vi "Begin Swerve Drive.vi"   [LabVIEW 2018]
uses:
  <vilib>/Rock Robotics/SystemInterfaces/DIO/FPGA_DIOPWMChannel.ctl
  <vilib>/Rock Robotics/SystemInterfaces/AI/FPGA_AIChannel.ctl
  <vilib>/Rock Robotics/SystemInterfaces/DIO/FPGA_DIOChannel.ctl
  <vilib>/Rock Robotics/WPI/RobotDrive/WPI_RobotDriveOpen4MotorWithTalon.vi
  <vilib>/Rock Robotics/WPI/Counter/WPI_CounterDigitalInputToDigitalSource.vi
types:
  T1 = typedef "FPGA_DIOChannel.ctl" = enum8{"DIO 0", "DIO 1", "DIO 2", "DIO 3", "DIO 4", "DIO 5", "DIO 6", "DIO 7", "DIO 8", "DIO 9", "DIO MXP 0", "DIO MXP 1", "DIO MXP 2", "DIO MXP 3", "DIO MXP 4", "DIO MXP 5", "DIO MXP 6", "DIO MXP 7", "DIO MXP 8", "DIO MXP 9", "DIO MXP 10", "DIO MXP 11", "DIO MXP 12", "DIO MXP 13", "DIO MXP 14", "DIO MXP 15", "SPI Port CS1", "SPI Port CS2", "SPI Port CS3", "SPI Port MISO", "SPI Port MOSI", "Invalid"}
  T2 = typedef "FPGA_AIChannel.ctl" = enum8{"AI 0", "AI 1", "AI 2", "AI 3", "AI MXP 0", "AI MXP 1", "AI MXP 2", "AI MXP 3", "Invalid"}
  T3 = typedef "FPGA_DIOPWMChannel.ctl" = enum8{"PWM 0", "PWM 1", "PWM 2", "PWM 3", "PWM 4", "PWM 5", "PWM 6", "PWM 7", "PWM 8", "PWM 9", "PWM MXP 0", "PWM MXP 1", "PWM MXP 2", "PWM MXP 3", "PWM MXP 4", "PWM MXP 5", "PWM MXP 6", "PWM MXP 7", "PWM MXP 8", "PWM MXP 9", "Invalid"}
  T4 = typedef "WPI_RobotDriveDevRef.ctl" = cluster{"DevStatus":errorcluster, "Motors[]":T5[], "Square Inputs":bool, "Max Output":dbl}
  T5 = typedef "WPI_MotorControlDeviceRef.ctl" = cluster{"DeviceStatus":errorcluster, "Type":T6, "PWM":cluster{"PWM Channel":T3, "DeadBand":T7}, "CAN":cluster{"Device Number":u8, "SetOutput VI Ref":variant, "GetOutput VI Ref":variant, "Enable VI Ref":variant, "Disable VI Ref":variant, "Data":variant}, "Invert":bool, "DIO PWM":cluster{"PWM \"Enable\" Channel":T3, "DIOChannel":T1, "PWM Rate":dbl}}
  T6 = typedef "WPI_MotorControlType.ctl" = enum16{"PWM", "CAN", "DIO PWM"}
  T7 = typedef "WPI_PWMDeadband.ctl" = cluster{"Name":string, "maxPositivePwm":i32, "minPositivePwm":i32, "centerPwm":i32, "maxNegativePwm":i32, "minNegativePwm":i32, "angularRange":u16}
  T8 = typedef "WPI_AnalogChannelDevRef.ctl" = cluster{"DevStatus":errorcluster, "Analog Channel":T2}
  T9 = typedef "WPI_DigitalInputDevRef.ctl" = cluster{"DevStatus":errorcluster, "DIO Channel":T1}
  T10 = typedef "FPGA_CounterEncoderSourceConvertionLVSourceType.ctl" = cluster{"DevStatus":errorcluster, "AnalogTriggerMode?":bool, "DigitalMode":cluster{"DIO Channel":T11}, "AnalogTriggerMode":cluster{"AnalogTriggerIndex":T12, "OutputType":T13}}
  T11 = typedef "FPGA_DIODigitalSourceChannel.ctl" = enum8{"DIO 0", "DIO 1", "DIO 2", "DIO 3", "DIO 4", "DIO 5", "DIO 6", "DIO 7", "DIO 8", "DIO 9", "DIO MXP 0", "DIO MXP 1", "DIO MXP 2", "DIO MXP 3", "DIO MXP 4", "DIO MXP 5", "DIO MXP 6", "DIO MXP 7", "DIO MXP 8", "DIO MXP 9", "DIO MXP 10", "DIO MXP 11", "DIO MXP 12", "DIO MXP 13", "DIO MXP 14", "DIO MXP 15", "SPI Port CS1", "SPI Port CS2", "SPI Port CS3", "SPI Port MISO", "SPI Port MOSI", "Disabled"}
  T12 = typedef "FPGA_AnalogTriggerIndex.ctl" = enum8{"Trig 0", "Trig 1", "Trig 2", "Trig 3", "Trig 4", "Trig 5", "Trig 6", "Trig 7", "Invalid"}
  T13 = typedef "FPGA_AnalogTriggerOutType.ctl" = enum16{"InWindow", "TriggerState", "Rising", "Falling"}
  T14 = typedef "WPI_EncoderDevRef.ctl" = cluster{"DevStatus":errorcluster, "EncoderIndex":T15, "CounterIndex":T16, "DistancePerCount":dbl, "Decoding Type":T17}
  T15 = typedef "FPGA_EncoderIdx.ctl" = enum8{"Enc 0", "Enc 1", "Enc 2", "Enc 3", "Enc 4", "Enc 5", "Enc 6", "Enc 7", "Invalid"}
  T16 = typedef "FPGA_CounterCtrSystemIndex.ctl" = enum8{"Ctr 0", "Ctr 1", "Ctr 2", "Ctr 3", "Ctr 4", "Ctr 5", "Ctr 6", "Ctr 7", "Invalid"}
  T17 = typedef "WPI_EncoderType.ctl" = enum16{"1x", "2x", "4x"}
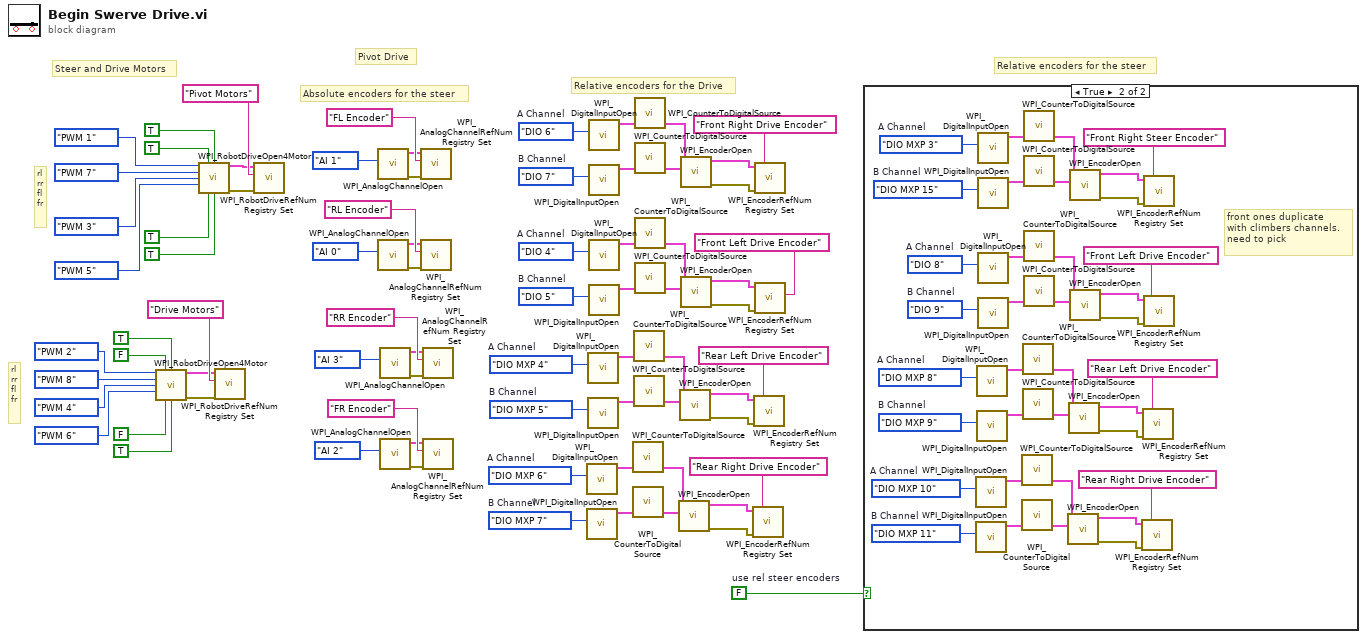
[diagram p0: block diagram]
diagram:
  w1 = FALSE  # use rel steer encoders
  w10 = FPGA_DIOChannel."DIO MXP 7"  # B Channel
  w9 = FPGA_DIOChannel."DIO MXP 6"  # A Channel
  w19 = FPGA_DIOChannel."DIO MXP 5"  # B Channel
  w18 = FPGA_DIOChannel."DIO MXP 4"  # A Channel
  w28 = FPGA_DIOChannel."DIO 5"  # B Channel
  w27 = FPGA_DIOChannel."DIO 4"  # A Channel
  w37 = FPGA_DIOChannel."DIO 7"  # B Channel
  w36 = FPGA_DIOChannel."DIO 6"  # A Channel
  # "Steer and Drive Motors"
  # "Absolute encoders for the steer"
  # "Relative encoders for the Drive"
  # "Relative encoders for the steer"
  # "Pivot Drive"
  # "rl\nrr\nfl\nfr"
  # "rl\nrr\nfl\nfr"
  n1 = call-poly <vilib>:"WPI_RobotDriveOpen4Motor.vi"("Rear Left Motor"=FPGA_DIOPWMChannel."PWM 2", "Rear Left Motor Inverted"=FALSE, "Rear Right Motor Inverted"=TRUE, "Rear Right Motor"=FPGA_DIOPWMChannel."PWM 8", "Front Left Motor"=FPGA_DIOPWMChannel."PWM 4", "Front Right Motor"=FPGA_DIOPWMChannel."PWM 6", "Front Left Motor Inverted"=FALSE, "Front Right Motor Inverted"=TRUE) -> ("RobotDriveDevRef"=w50:T4, "error out"=w49:errorcluster)  [unwired: 6 in]
  n2 = call-poly <vilib>:"WPI_RobotDriveOpen4Motor.vi"("Rear Left Motor"=FPGA_DIOPWMChannel."PWM 1", "Rear Left Motor Inverted"=TRUE, "Rear Right Motor Inverted"=TRUE, "Rear Right Motor"=FPGA_DIOPWMChannel."PWM 7", "Front Left Motor"=FPGA_DIOPWMChannel."PWM 3", "Front Right Motor"=FPGA_DIOPWMChannel."PWM 5", "Front Left Motor Inverted"=TRUE, "Front Right Motor Inverted"=TRUE) -> ("RobotDriveDevRef"=w39:T4, "error out"=w38:errorcluster)  [unwired: 6 in]
  n3 = call <vilib>:"WPI_RobotDriveRefNum Registry Set.vi"("error in (no error)"=w49, "refnum name"="Drive Motors", "RobotDriveDevRef"=w50) -> ()  [unwired: 7 in, 2 out]
  n4 = call <vilib>:"WPI_RobotDriveRefNum Registry Set.vi"("error in (no error)"=w38, "refnum name"="Pivot Motors", "RobotDriveDevRef"=w39) -> ()  [unwired: 7 in, 2 out]
  n5 = call <vilib>:"WPI_AnalogChannelOpen.vi"("Analog Channel"=FPGA_AIChannel."AI 1") -> ("error out"=w64:errorcluster, "AIDeviceRef"=w65:T8)  [unwired: 9 in]
  n6 = call <vilib>:"WPI_AnalogChannelOpen.vi"("Analog Channel"=FPGA_AIChannel."AI 0") -> ("error out"=w60:errorcluster, "AIDeviceRef"=w61:T8)  [unwired: 9 in]
  n7 = call <vilib>:"WPI_AnalogChannelOpen.vi"("Analog Channel"=FPGA_AIChannel."AI 3") -> ("error out"=w72:errorcluster, "AIDeviceRef"=w73:T8)  [unwired: 9 in]
  n8 = call <vilib>:"WPI_AnalogChannelOpen.vi"("Analog Channel"=FPGA_AIChannel."AI 2") -> ("error out"=w68:errorcluster, "AIDeviceRef"=w69:T8)  [unwired: 9 in]
  n9 = call <vilib>:"WPI_AnalogChannelRefNum Registry Set.vi"("error in (no error)"=w64, "refnum name"="FL Encoder", "AIDeviceRef"=w65) -> ()  [unwired: 7 in, 2 out]
  n10 = call <vilib>:"WPI_AnalogChannelRefNum Registry Set.vi"("error in (no error)"=w60, "refnum name"="RL Encoder", "AIDeviceRef"=w61) -> ()  [unwired: 7 in, 2 out]
  n11 = call <vilib>:"WPI_AnalogChannelRefNum Registry Set.vi"("error in (no error)"=w72, "refnum name"="RR Encoder", "AIDeviceRef"=w73) -> ()  [unwired: 7 in, 2 out]
  n12 = call <vilib>:"WPI_AnalogChannelRefNum Registry Set.vi"("error in (no error)"=w68, "refnum name"="FR Encoder", "AIDeviceRef"=w69) -> ()  [unwired: 7 in, 2 out]
  n13 = call <vilib>:"WPI_DigitalInputOpen.vi"("DIO Channel"=w9) -> ("DigitalInputDevRef"=w6:T9)  [unwired: 1 in, 9 out]
  n14 = call <vilib>:"WPI_DigitalInputOpen.vi"("DIO Channel"=w10) -> ("DigitalInputDevRef"=w7:T9)  [unwired: 1 in, 9 out]
  n15 = call <vilib>:"WPI_DigitalInputOpen.vi"("DIO Channel"=w18) -> ("DigitalInputDevRef"=w15:T9)  [unwired: 1 in, 9 out]
  n16 = call <vilib>:"WPI_DigitalInputOpen.vi"("DIO Channel"=w19) -> ("DigitalInputDevRef"=w16:T9)  [unwired: 1 in, 9 out]
  n17 = call <vilib>:"WPI_DigitalInputOpen.vi"("DIO Channel"=w36) -> ("DigitalInputDevRef"=w33:T9)  [unwired: 1 in, 9 out]
  n18 = call <vilib>:"WPI_DigitalInputOpen.vi"("DIO Channel"=w37) -> ("DigitalInputDevRef"=w34:T9)  [unwired: 1 in, 9 out]
  n19 = call <vilib>:"WPI_DigitalInputOpen.vi"("DIO Channel"=w27) -> ("DigitalInputDevRef"=w24:T9)  [unwired: 1 in, 9 out]
  n20 = call <vilib>:"WPI_DigitalInputOpen.vi"("DIO Channel"=w28) -> ("DigitalInputDevRef"=w25:T9)  [unwired: 1 in, 9 out]
  n21 = call-poly <vilib>:"WPI_CounterToDigitalSource.vi"("DigitalInputDevRef"=w6) -> ("Digital Source"=w5:T10)  [unwired: 6 out]
  n22 = call-poly <vilib>:"WPI_CounterToDigitalSource.vi"("DigitalInputDevRef"=w7) -> ("Digital Source"=w8:T10)  [unwired: 6 out]
  n23 = call-poly <vilib>:"WPI_CounterToDigitalSource.vi"("DigitalInputDevRef"=w15) -> ("Digital Source"=w14:T10)  [unwired: 6 out]
  n24 = call-poly <vilib>:"WPI_CounterToDigitalSource.vi"("DigitalInputDevRef"=w16) -> ("Digital Source"=w17:T10)  [unwired: 6 out]
  n25 = call-poly <vilib>:"WPI_CounterToDigitalSource.vi"("DigitalInputDevRef"=w33) -> ("Digital Source"=w32:T10)  [unwired: 6 out]
  n26 = call-poly <vilib>:"WPI_CounterToDigitalSource.vi"("DigitalInputDevRef"=w34) -> ("Digital Source"=w35:T10)  [unwired: 6 out]
  n27 = call-poly <vilib>:"WPI_CounterToDigitalSource.vi"("DigitalInputDevRef"=w24) -> ("Digital Source"=w23:T10)  [unwired: 6 out]
  n28 = call-poly <vilib>:"WPI_CounterToDigitalSource.vi"("DigitalInputDevRef"=w25) -> ("Digital Source"=w26:T10)  [unwired: 6 out]
  n29 = call <vilib>:"WPI_EncoderOpen.vi"("BSource"=w8, "ASource"=w5) -> ("error out"=w3:errorcluster, "EncoderDevRef"=w4:T14)  [unwired: 6 in, 2 out]
  n30 = call <vilib>:"WPI_EncoderOpen.vi"("BSource"=w17, "ASource"=w14) -> ("error out"=w12:errorcluster, "EncoderDevRef"=w13:T14)  [unwired: 6 in, 2 out]
  n31 = call <vilib>:"WPI_EncoderOpen.vi"("BSource"=w35, "ASource"=w32) -> ("error out"=w30:errorcluster, "EncoderDevRef"=w31:T14)  [unwired: 6 in, 2 out]
  n32 = call <vilib>:"WPI_EncoderOpen.vi"("BSource"=w26, "ASource"=w23) -> ("error out"=w21:errorcluster, "EncoderDevRef"=w22:T14)  [unwired: 6 in, 2 out]
  n33 = call <vilib>:"WPI_EncoderRefNum Registry Set.vi"("error in (no error)"=w3, "refnum name"="Rear Right Drive Encoder", "EncoderDevRef"=w4) -> ()  [unwired: 7 in, 2 out]
  n34 = call <vilib>:"WPI_EncoderRefNum Registry Set.vi"("error in (no error)"=w12, "refnum name"="Rear Left Drive Encoder", "EncoderDevRef"=w13) -> ()  [unwired: 7 in, 2 out]
  n35 = call <vilib>:"WPI_EncoderRefNum Registry Set.vi"("error in (no error)"=w30, "refnum name"="Front Right Drive Encoder", "EncoderDevRef"=w31) -> ()  [unwired: 7 in, 2 out]
  n36 = call <vilib>:"WPI_EncoderRefNum Registry Set.vi"("error in (no error)"=w21, "refnum name"="Front Left Drive Encoder", "EncoderDevRef"=w22) -> ()  [unwired: 7 in, 2 out]
  n37 = case shown="True" w1 {
    frame False {
    }
    frame True {
      w103 = FPGA_DIOChannel."DIO MXP 11"  # B Channel
      w104 = FPGA_DIOChannel."DIO MXP 10"  # A Channel
      w94 = FPGA_DIOChannel."DIO MXP 9"  # B Channel
      w95 = FPGA_DIOChannel."DIO MXP 8"  # A Channel
      w85 = FPGA_DIOChannel."DIO 9"  # B Channel
      w86 = FPGA_DIOChannel."DIO 8"  # A Channel
      w76 = FPGA_DIOChannel."DIO MXP 15"  # B Channel
      w77 = FPGA_DIOChannel."DIO MXP 3"  # A Channel
      # "front ones duplicate\nwith climbers channels.\nneed to pick"
      n38 = call <vilib>:"WPI_DigitalInputOpen.vi"("DIO Channel"=w104) -> ("DigitalInputDevRef"=w107:T9)  [unwired: 1 in, 9 out]
      n39 = call <vilib>:"WPI_DigitalInputOpen.vi"("DIO Channel"=w103) -> ("DigitalInputDevRef"=w106:T9)  [unwired: 1 in, 9 out]
      n40 = call <vilib>:"WPI_DigitalInputOpen.vi"("DIO Channel"=w95) -> ("DigitalInputDevRef"=w98:T9)  [unwired: 1 in, 9 out]
      n41 = call <vilib>:"WPI_DigitalInputOpen.vi"("DIO Channel"=w94) -> ("DigitalInputDevRef"=w97:T9)  [unwired: 1 in, 9 out]
      n42 = call <vilib>:"WPI_DigitalInputOpen.vi"("DIO Channel"=w77) -> ("DigitalInputDevRef"=w80:T9)  [unwired: 1 in, 9 out]
      n43 = call <vilib>:"WPI_DigitalInputOpen.vi"("DIO Channel"=w76) -> ("DigitalInputDevRef"=w79:T9)  [unwired: 1 in, 9 out]
      n44 = call <vilib>:"WPI_DigitalInputOpen.vi"("DIO Channel"=w86) -> ("DigitalInputDevRef"=w89:T9)  [unwired: 1 in, 9 out]
      n45 = call <vilib>:"WPI_DigitalInputOpen.vi"("DIO Channel"=w85) -> ("DigitalInputDevRef"=w88:T9)  [unwired: 1 in, 9 out]
      n46 = call-poly <vilib>:"WPI_CounterToDigitalSource.vi"("DigitalInputDevRef"=w107) -> ("Digital Source"=w108:T10)  [unwired: 6 out]
      n47 = call-poly <vilib>:"WPI_CounterToDigitalSource.vi"("DigitalInputDevRef"=w106) -> ("Digital Source"=w105:T10)  [unwired: 6 out]
      n48 = call-poly <vilib>:"WPI_CounterToDigitalSource.vi"("DigitalInputDevRef"=w98) -> ("Digital Source"=w99:T10)  [unwired: 6 out]
      n49 = call-poly <vilib>:"WPI_CounterToDigitalSource.vi"("DigitalInputDevRef"=w97) -> ("Digital Source"=w96:T10)  [unwired: 6 out]
      n50 = call-poly <vilib>:"WPI_CounterToDigitalSource.vi"("DigitalInputDevRef"=w80) -> ("Digital Source"=w81:T10)  [unwired: 6 out]
      n51 = call-poly <vilib>:"WPI_CounterToDigitalSource.vi"("DigitalInputDevRef"=w79) -> ("Digital Source"=w78:T10)  [unwired: 6 out]
      n52 = call-poly <vilib>:"WPI_CounterToDigitalSource.vi"("DigitalInputDevRef"=w89) -> ("Digital Source"=w90:T10)  [unwired: 6 out]
      n53 = call-poly <vilib>:"WPI_CounterToDigitalSource.vi"("DigitalInputDevRef"=w88) -> ("Digital Source"=w87:T10)  [unwired: 6 out]
      n54 = call <vilib>:"WPI_EncoderOpen.vi"("BSource"=w105, "ASource"=w108) -> ("error out"=w110:errorcluster, "EncoderDevRef"=w109:T14)  [unwired: 6 in, 2 out]
      n55 = call <vilib>:"WPI_EncoderOpen.vi"("BSource"=w96, "ASource"=w99) -> ("error out"=w101:errorcluster, "EncoderDevRef"=w100:T14)  [unwired: 6 in, 2 out]
      n56 = call <vilib>:"WPI_EncoderOpen.vi"("BSource"=w78, "ASource"=w81) -> ("error out"=w83:errorcluster, "EncoderDevRef"=w82:T14)  [unwired: 6 in, 2 out]
      n57 = call <vilib>:"WPI_EncoderOpen.vi"("BSource"=w87, "ASource"=w90) -> ("error out"=w92:errorcluster, "EncoderDevRef"=w91:T14)  [unwired: 6 in, 2 out]
      n58 = call <vilib>:"WPI_EncoderRefNum Registry Set.vi"("error in (no error)"=w110, "refnum name"="Rear Right Drive Encoder", "EncoderDevRef"=w109) -> ()  [unwired: 7 in, 2 out]
      n59 = call <vilib>:"WPI_EncoderRefNum Registry Set.vi"("error in (no error)"=w101, "refnum name"="Rear Left Drive Encoder", "EncoderDevRef"=w100) -> ()  [unwired: 7 in, 2 out]
      n60 = call <vilib>:"WPI_EncoderRefNum Registry Set.vi"("error in (no error)"=w83, "refnum name"="Front Right Steer Encoder", "EncoderDevRef"=w82) -> ()  [unwired: 7 in, 2 out]
      n61 = call <vilib>:"WPI_EncoderRefNum Registry Set.vi"("error in (no error)"=w92, "refnum name"="Front Left Drive Encoder", "EncoderDevRef"=w91) -> ()  [unwired: 7 in, 2 out]
    }
  }
